vi "Simple Scale.vi"() -> ()   [LabVIEW 2023]
doc: "Uses the Calc Scale Specs VI and the Draw Scale VI to draw a scale of a Cartesian graph in a picture indicator. You can change the range, location, and orientation of the scale."
panel:
  in  "Scale Definition":T1={"Starting Position"=10, "Starting Value"=0.0, "Ending Position"=100, "Ending Value"=10.0, "Log?"=FALSE, "Format and Precision"={"Format"=0, "Precision"=0}} {"Format and Precision"."Format" items=["Decimal", "Scientific", "Engineering", "Binary", "Octal", "Hex"]}
  in  "Scalar Attributes":T2={"Horizontal"=FALSE, "Left/Top"=TRUE, "Draw Bar"=TRUE, "Line Color"=16726058, "Text Color"=0}
  in  "Constant Coordinate":i16=100
  out "Picture":picture
  # "Overview: Uses the Calc Scale Specs VI and the Draw Scale VI to draw a scale of a Cartesian graph in a picture indicator.\nInstructions:\n1. Run the VI.\n2. Modify the Scalar Attributes and Scale Definition controls to change how the scale is displayed."
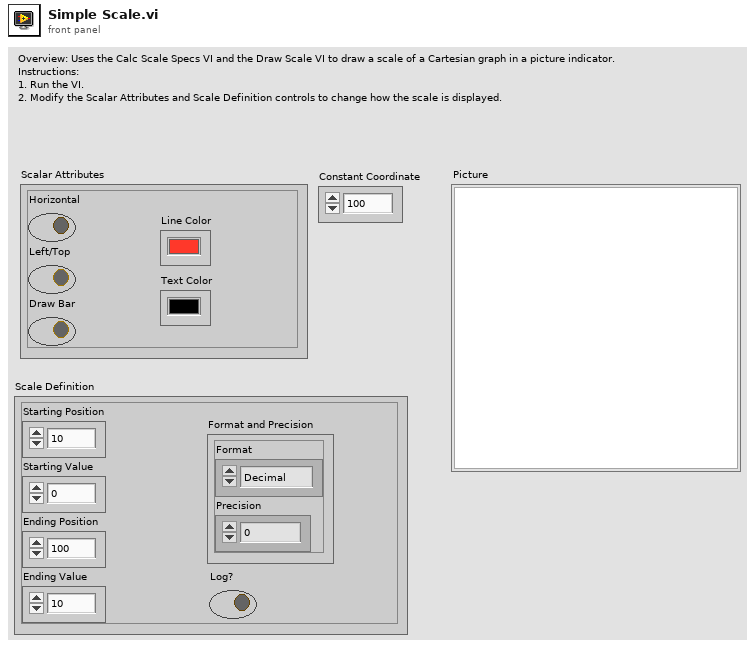
[diagram p1: front panel]
types:
  T1 = cluster{"Starting Position":i16, "Starting Value":dbl, "Ending Position":i16, "Ending Value":dbl, "Log?":bool, "Format and Precision":cluster{"Format":u16, "Precision":u8}}
  T2 = cluster{"Horizontal":bool, "Left/Top":bool, "Draw Bar":bool, "Line Color":u32, "Text Color":u32}
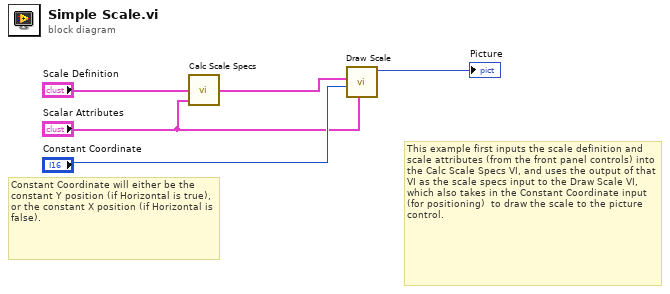
[diagram p0: block diagram]
diagram:
  # "This example first inputs the scale definition and scale attributes (from the front panel controls) into the Calc Scale Specs VI, and uses the output of that VI as the scale specs input to the Draw Scale VI, which also takes in the Constant Coordinate input (for positioning)  to draw the scale to the picture control."
  # "Constant Coordinate will either be the constant Y position (if Horizontal is true), or the constant X position (if Horizontal is false)."
  n1 = call <vilib>:"Calc Scale Specs.vi"("scale definition"="Scale Definition", "scale attributes"="Scalar Attributes") -> ("scale specs"=w1:cluster{"coordinate":i16, "label":string}[])  [unwired: 7 in]
  n2 = call <vilib>:"Draw Scale.vi"("scale attributes"="Scalar Attributes", "constant coordinate"="Constant Coordinate", "scale specs"=w1) -> ("new picture"=→"Picture":picture)  [unwired: 8 in]
